vi "SeCrTs-ACC_Scale_Config.vi"(8 "error in (no error)":errorcluster, 10 "ACC config":T1(array[cluster]), 11 "Refnum in":refnum<k21>) -> (0 "error out":errorcluster, 3 "Refnum out":refnum<k21>)   [LabVIEW 2022 SP3]
uses:
  <vilib>/DAQmx/create/channels.llb/DAQmx Create Channel (AI-Acceleration-Accelerometer).vi
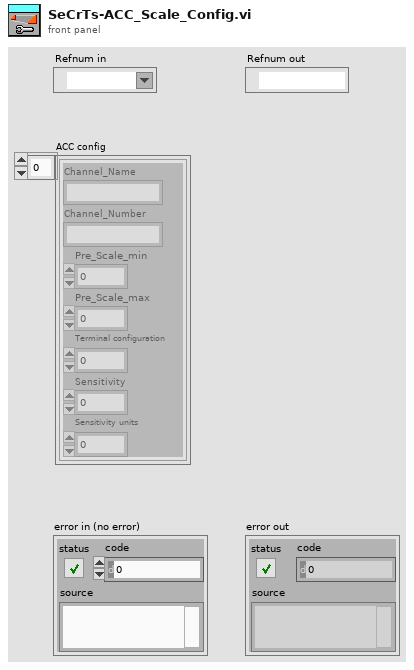
[diagram p1: front panel]
types:
  T1 = cluster{"Channel_Name":string, "Channel_Number":string, "Pre_Scale_min":dbl, "Pre_Scale_max":dbl, "Terminal configuration":i32, "Sensitivity":dbl, "Sensitivity units":i32}[]
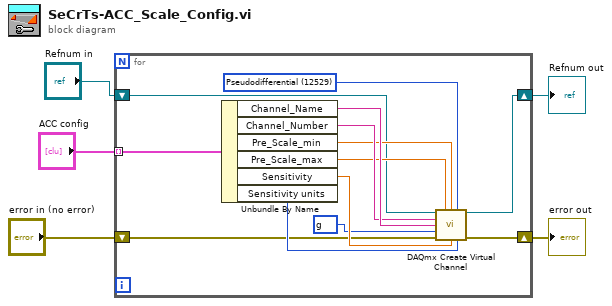
[diagram p0: block diagram]
diagram:
  n1 = for {
    tunnel: "ACC config" -> [w18] mode=indexing
    shift-right: [w10] -> w2
    shift-left: "error in (no error)" -> [w9]
    shift-right: [w11] -> w3
    shift-left: "Refnum in" -> [w7]
    w6 = 10186 items=["g"=10186, "m/s^2"=12470, "in/s^2"=12471, "From Custom Scale"=10065] ("units")
    w8 = 12529 items=["default"=-1, "RSE"=10083, "NRSE"=10078, "Differential"=10106, "Pseudodifferential"=12529] ("input terminal configuration")
    n2 = Unbundle By Name(w18) -> ("Channel_Name"=w17:string, "Channel_Number"=w16:string, "Pre_Scale_min"=w13:dbl, "Pre_Scale_max"=w12:dbl, "Sensitivity"=w14:dbl, "Sensitivity units"=w15:i32)
    n3 = call-poly <vilib>:"DAQmx Create Virtual Channel.vi"("task in"=w7, "maximum value"=w12, "minimum value"=w13, "input terminal configuration"=w8, "physical channels"=w16, "name to assign"=w17, "units"=w6, "error in"=w9, "sensitivity"=w14, "sensitivity units"=w15) -> ("task out"=w11:refnum<k21>, "error out"=w10:errorcluster)  [unwired: 4 in]
  }
  "Refnum out" <- w3
  "error out" <- w2
